vi "Set Flexible Size.vi"(8 "error in (no error)":errorcluster, 9 "Max Size (1024x768)":cluster{"Width":i32, "Height":i32}={"Width"=1024, "Height"=768}, 10 "Flexible?":bool, 11 "Dialog in":refnum<class "Dialog.lvclass">) -> (0 "error out":errorcluster, 3 "Dialog out":refnum<class "Dialog.lvclass">)   [LabVIEW 2012, in "Dialog.lvlib" / "Dialog.lvclass"]
uses:
  Dialog.lvclass
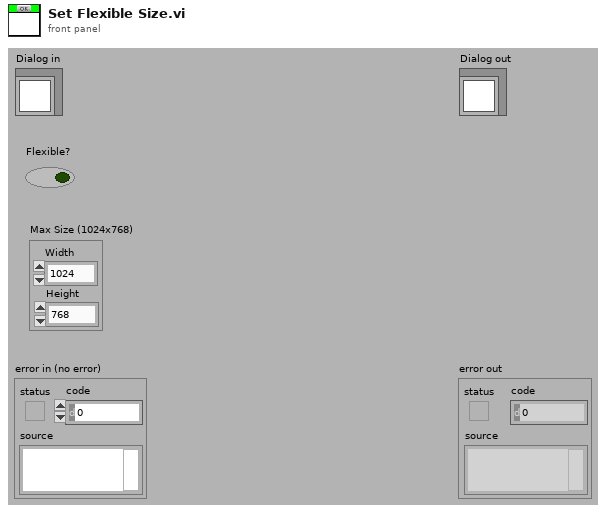
[diagram p1: front panel]
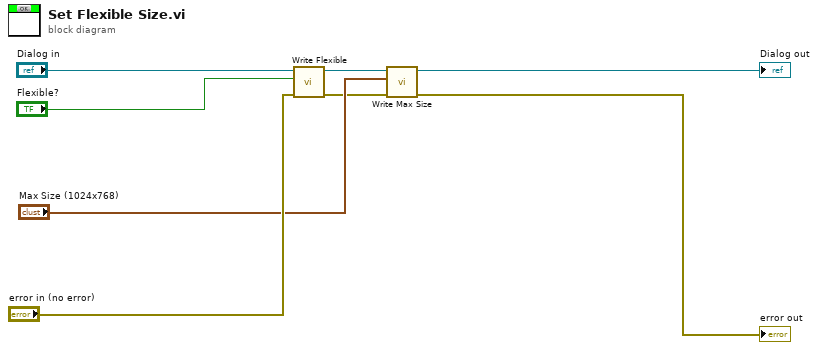
[diagram p0: block diagram]
diagram:
  n1 = call-dynamic "Write Flexible.vi"("error in (no error)"="error in (no error)", "flexible?"="Flexible?", "Dialog.lvclass in"="Dialog in") -> ("error out"=w1:errorcluster, "Dialog.lvclass out"=w2:refnum<class "Dialog.lvclass">)  [unwired: 7 out]
  n2 = call-dynamic "Write Max Size.vi"("error in (no error)"=w1, "Max Size"="Max Size (1024x768)", "Dialog.lvclass in"=w2) -> ("error out"=→"error out":errorcluster, "Dialog.lvclass out"=→"Dialog out":refnum<class "Dialog.lvclass">)  [unwired: 7 out]
